vi "LiCor_init.vi"(1 "VISA resource name":refnum<visa-resource-name>="COM1") -> (0 "LiCor session out":T1={"VISA resource out"="COM12", "error out"={"status"=FALSE, "code"=0, "source"=""}})   [LabVIEW 2010]
uses:
  <vilib>/Instr/_visa.llb/VISA Configure Serial Port (Instr).vi
panel:
  # "This VI simply does the initialization work of setting the Li-Cor VISA resource with all the settings that seems to work. It passes out a VISA out and error out line for passing through the flow of the rest of the applications in which it may be used."
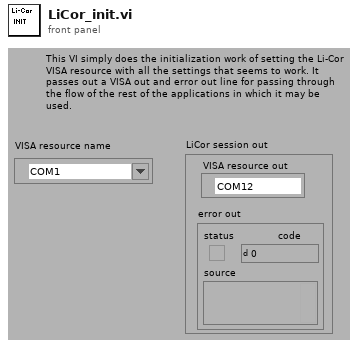
[diagram p1: front panel]
types:
  T1 = cluster{"VISA resource out":refnum<visa-resource-name>, "error out":errorcluster}
  T2 = cluster{"VISA resource name out":refnum<visa-resource-name>, "error out":errorcluster}
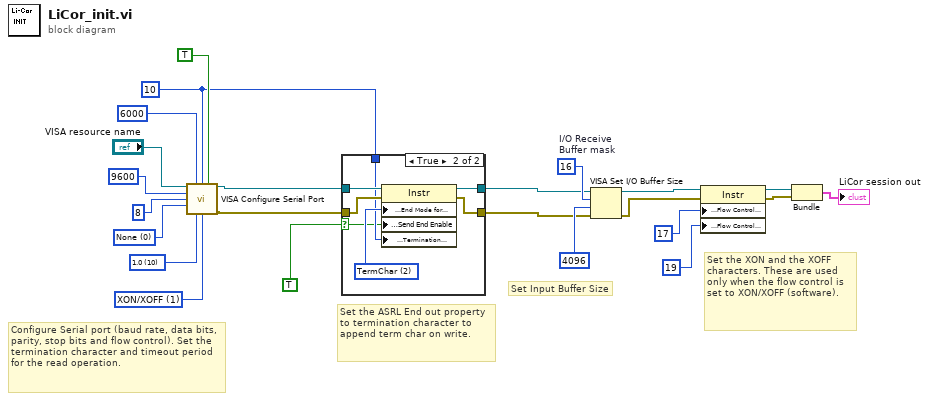
[diagram p0: block diagram]
diagram:
  w13 = u16 1 items=["None"=0, "XON/XOFF"=1, "RTS/CTS"=2, "DTR/DSR"=4] ("flow control")
  w20 = u16 10 items=["1.0"=10, "1.5"=15, "2.0"=20] ("stop bits")
  w21 = u16 0 items=["None", "Odd", "Even", "Mark", "Space"] ("parity")
  w14 = u8 10 ("termination char\n(0xA = '\\n' = LF)")
  w17 = u16 16  # I/O Receive Buffer mask
  # "Set the XON and the XOFF characters. These are used only when the flow control is set to XON/XOFF (software)."
  # "Configure Serial port (baud rate, data bits, parity, stop bits and flow control). Set the termination character and timeout period for the read operation."
  # "Set Input Buffer Size"
  # "Set the ASRL End out property to termination character to append term char on write."
  n1 = call-poly "VISA Configure Serial Port"("VISA resource name"="VISA resource name", "timeout (10sec)"=u32 6000 ("timeout (ms)"), "termination char\n(0xA = '\\n' = LF)"=w14, "Enable Termination\nChar (T)"=TRUE ("End read on termination character?"), "baud rate (9600)"=u32 9600 ("baud rate"), "data bits (8)"=u16 8 ("data bits"), "parity (0:none)"=w21, "stop bits (10: 1 bit)"=w20, "flow control (0:none)"=w13) -> ("VISA resource name out"=w5:refnum<visa-resource-name>, "error out"=w4:errorcluster)  [unwired: 1 in, 4 out]
  n2 = case shown="True" TRUE ("End write with termination character?") {
    selector: TRUE ("End write with termination character?") -> [_ w26]
    tunnel: w5 -> [w24 w32]
    tunnel: w4 -> [w25 w31]
    tunnel: [w24 w30] -> w6
    tunnel: [w25 w29] -> w7
    tunnel: w14 -> [_ w27]
    frame False {
    }
    frame True {
      w28 = u16 2 items=["None", "LastBit", "TermChar", "Break"] ("Serial Settings:Serial End Mode for Writes")
      n3 = property class="Instr"(reference=w32, error in=w31, "Serial Settings:End Mode for Writes"=w28, "Message Based Settings:Send End Enable"=w26, "Message Based Settings:Termination Character"=w27) -> (reference out=w30:refnum<visa-resource-name>, error out=w29:errorcluster)
    }
  }
  n4 = VISA Set I/O Buffer Size(VISA resource name=w6, mask (16)=w17, size (4096)=u32 4096 ("Input\nbuffer size"), error in (no error)=w7) -> (VISA resource name out=w12:refnum<visa-resource-name>, error out=w11:errorcluster)
  n5 = property class="Instr"(reference=w12, error in=w11, "Serial Settings:Flow Control XON Character"=u8 17 ("XON Character"), "Serial Settings:Flow Control XOFF Character"=u8 19 ("XOFF Character")) -> (reference out=w3:refnum<visa-resource-name>, error out=w2:errorcluster)
  n6 = Bundle("VISA resource name out"=w3, "error out"=w2) -> (→"LiCor session out":T2)  [unwired: 1 in]
